vi "GMU2 Channel Names.vi"() -> (2 "GMU2 Source Channels":string[](array[string])=["GMU2:Source Carrier:", "GMU2:Source Trace:"], 3 "GMU2 Calib Channels":string[](array[string])=["GMU2:Calib Carrier:", "GMU2:Calib Trace:"])   [LabVIEW 2022 SP3]
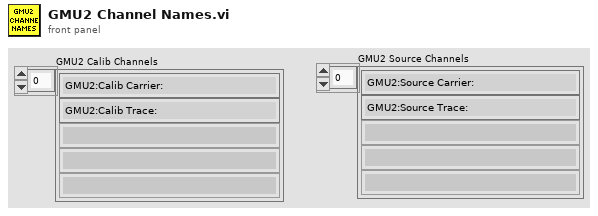
[diagram p1: front panel]
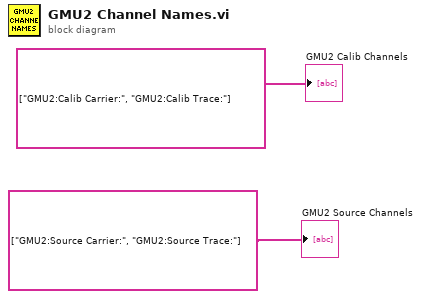
[diagram p0: block diagram]
diagram:
  "GMU2 Calib Channels" <- string[] ["GMU2:Calib Carrier:", "GMU2:Calib Trace:"] ("appended array")
  "GMU2 Source Channels" <- string[] ["GMU2:Source Carrier:", "GMU2:Source Trace:"] ("appended array")
